vi "Dashboard Main.vi"() -> ()   [LabVIEW 2017]
uses:
  <vilib>/Utility/miscctls.llb/LVRowAndColumnTypeDef.ctl
  <vilib>/event_ctls.llb/eventvkey.ctl
  <vilib>/Rock Robotics/Network Tables/NT Read Numeric Array.vi
  <vilib>/Utility/inputDevices.llb/keyboardAcquire.vi
  <vilib>/Utility/inputDevices.llb/closeKeyboard.vi
  <vilib>/Rock Robotics/WPI/Dashboard/WPI_DashboardLogging Global.vi
panel:
  out "Key Pressed":T1(array[ring])
  out "Key Pressed as String":string
  in  "Camera Settings Right":T2={"Frame Rate"=30, "Compression"=30, "Size"=1, "DB Camera Config"=FALSE} {"Frame Rate" scale=1.0..30.0; "Compression" scale=100.0..-1.0; "Size" items=["640x480", "320x240", "160x120"]}
  in  "Camera Name Right":string(combo)="No Camera Selection"
  out "Camera Info":cluster{"Mbps LED":bool, "Mbps":dbl, "fps":dbl} {"fps" format="%#.1g"; "Mbps" format="%#.1g"}
  in  "Camera Settings":T2={"Frame Rate"=30, "Compression"=30, "Size"=1, "DB Camera Config"=FALSE} {"Frame Rate" scale=1.0..30.0; "Compression" scale=100.0..-1.0; "Size" items=["640x480", "320x240", "160x120"]}
  in  "TCP":refnum<k5>
  in  "Rec Mode":enum32{"Stop", "Record", "Playback"}(radio)
  out "Robot IP":string
  out "Image Message":string="Timeout in Camera Communications"
  in  "Dashboard Tab":T3(tab)
  in  "Select Auto":string(combo)="Select Autonomous ..."
  out "NT Connection":bool
  out "MotorChart R":cluster{"Numeric":dbl, "Numeric":dbl}(graph)
  out "MotorChart L":cluster{"Numeric":dbl, "Numeric":dbl}(graph)
  out "MotorSliders R":cluster{"MotorSlide1":dbl, "MotorSlide2":dbl} {"MotorSlide2" scale=-1.0..1.0 scale format="%#_2e"; "MotorSlide1" scale=-1.0..1.0 scale format="%#_2e"}
  out "MotorSliders L":cluster{"MotorSlide1":dbl, "MotorSlide2":dbl} {"MotorSlide2" scale=-1.0..1.0 scale format="%#_2e"; "MotorSlide1" scale=-1.0..1.0 scale format="%#_2e"}
  out "Gyro":dbl(knob) scale=0.0..360.0
  out "JS1 Z":dbl(slide) scale=-1.0..1.0 scale format="%#_2e"
  out "JS1 Graph":cluster{"X":dbl, "Y":dbl}[](graph)
  out "JS1 Buttons":T4
  out "JS2 Z":dbl(slide) scale=-1.0..1.0 scale format="%#_2e"
  out "JS2 Graph":cluster{"X":dbl, "Y":dbl}[](graph)
  out "JS2 Buttons":T4
  out "Mode":T5(ring)=enum."Auto Disabled"
  out "Camera Image Right":T6(plugin-control)
  in  "DB/String 9":string
  in  "DB/String 8":string
  in  "DB/String 7":string
  in  "DB/String 6":string
  in  "DB/String 5":string
  in  "DB/String 4":string
  in  "DB/String 3":string
  in  "DB/String 2":string
  in  "DB/String 1":string
  in  "DB/String 0":string
  in  "DB/Slider 0":dbl(slide) scale=0.0..5.0
  in  "DB/Slider 1":dbl(slide) scale=0.0..5.0
  in  "DB/Slider 2":dbl(slide) scale=0.0..5.0
  in  "DB/Slider 3":dbl(slide) scale=0.0..5.0
  out "DB/LED 3":bool
  out "DB/LED 2":bool
  out "DB/LED 1":bool
  out "DB/LED 0":bool
  in  "DB/Button 3":bool
  in  "DB/Button 2":bool
  in  "DB/Button 1":bool
  in  "DB/Button 0":bool caption="New Name"
  in  "Test Slider":dbl(slide) scale=0.0..100.0 scale format="%#_3g"
  in  "On/Off":bool caption="Solenoid"
  in  "Test Name":u16(ring) items=["Select the test to run..."]
  in  "Test Tree":string(tree)
  in  "Motor":cluster{"Value":dbl, "Enable":bool} {"Value" scale=-1.0..1.0 scale format="%#_3g"}
  out "Progress":T7 {"Test Progress" scale=0.0..100.0}
  in  "Rev/Fwd":cluster{"Forward":bool, "Reverse":bool}
  in  "Test Ring":u16(ring) items=["Monochrome", "Color"]
  out "Cmd Status":string
  in  "Execute Command":bool
  in  "Command Params":string[][](table)
  in  "Command Selection":i32(listbox)
  in  "CheckList":i32(listbox)
  out "Tree":string(tree)
  out "Camera Image":T6(plugin-control)
  out "Background":bool
  in  "Camera Name":string(combo)="No Camera Selection"
  # "HW"
  # "HW"
  # "Joysticks"
  # "Drive Motors"
  # "Front"
  # "Right"
  # "Left"
  # "Back"
  # "This tab is a great place for autonomous settings and robot-specific values.\nPlace controls and indicators inside this tab and match name to\nDashboard Variables on robot. You can also delete this comment."
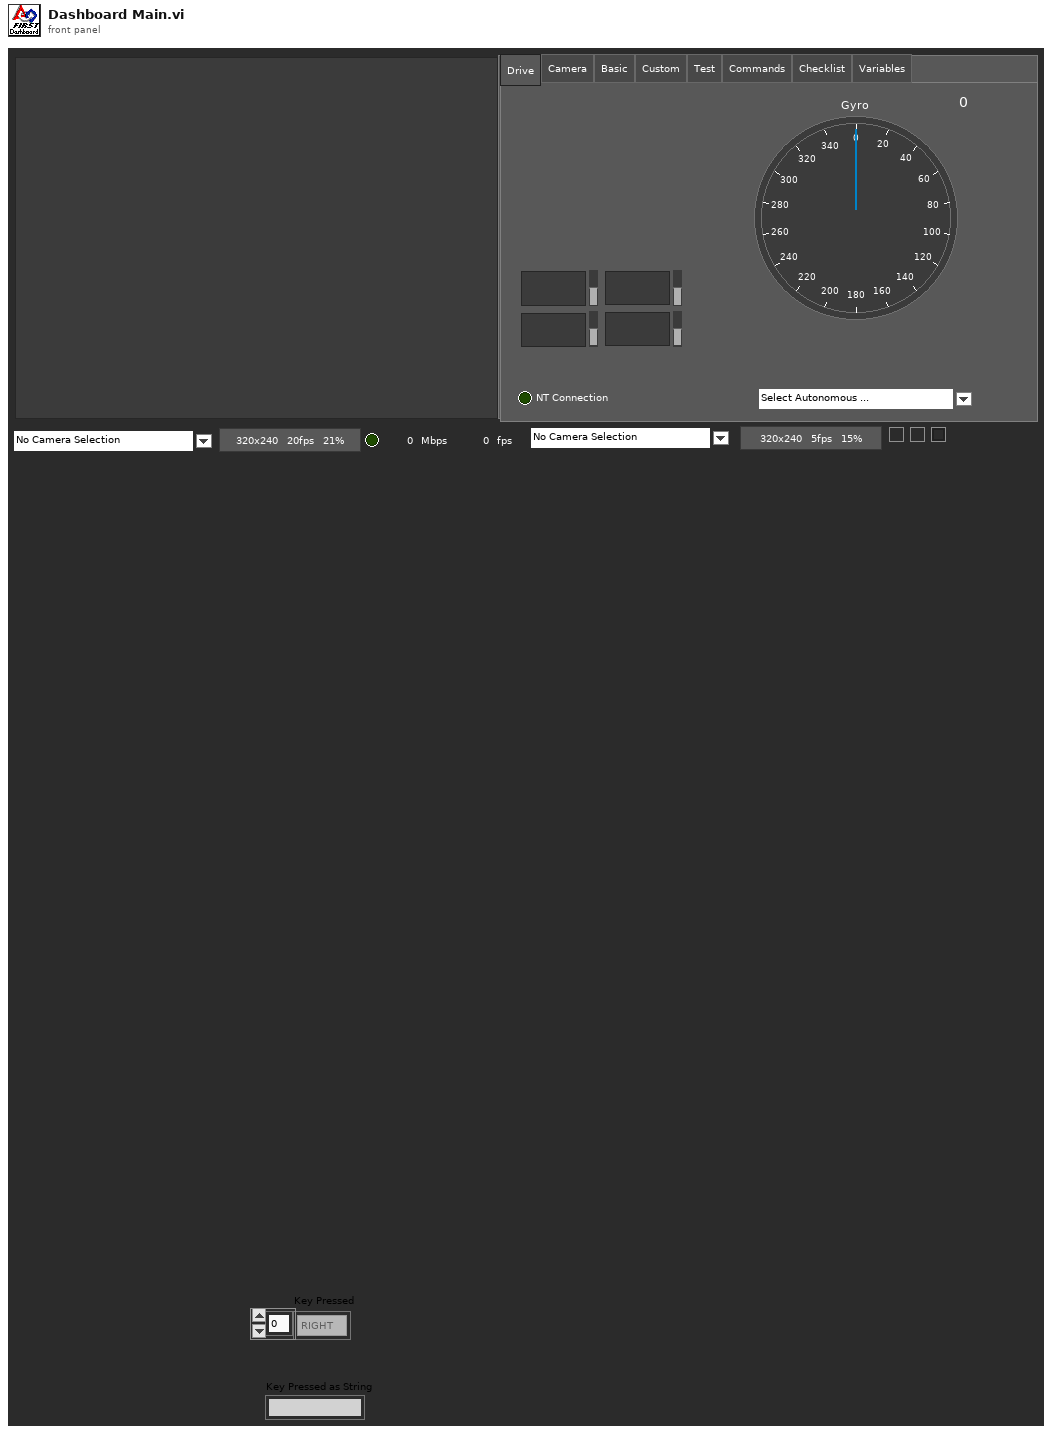
[diagram p1: front panel]
types:
  T1 = enum16{"0", "1", "2", "3", "4", "5", "6", "7", "8", "9", "A", "B", "C", "D", "E", "F", "G", "H", "I", "J", "K", "L", "M", "N", "O", "P", "Q", "R", "S", "T", "U", "V", "W", "X", "Y", "Z", "F1", "F2", "F3", "F4", "F5", "F6", "F7", "F8", "F9", "F10", "F11", "F12", "F13", "F14", "F15", "ADD", "BACK", "BACKSLASH", "CAPITAL", "COMMA", "DECIMAL", "DELETE", "DIVIDE", "DOWN", "END", "EQUALS", "ESCAPE", "GRAVE (`)", "HOME", "INSERT", "LBRACKET", "LCONTROL", "LEFT", "L ALT", "LSHIFT", "LWIN", "MINUS", "MULTIPLY", "NEXT", "NUMLOCK", "NUMPAD_0", "NUMPAD_1", "NUMPAD_2", "NUMPAD_3", "NUMPAD_4", "NUMPAD_5", "NUMPAD_6", "NUMPAD_7", "NUMPAD_8", "NUMPAD_9", "PAUSE", "PERIOD", "PRIOR (PG UP)", "RBRACKET", "RCONTROL", "RETURN", "RIGHT", "R ALT", "RSHIFT", "RWIN", "SCROLL", "SEMICOLON", "SLASH", "SPACE", "SUBTRACT", "TAB", "UP", "ENTER (num pad)", "' (quote)"}[]
  T2 = cluster{"Frame Rate":i32, "Compression":i32, "Size":u16, "DB Camera Config":bool}
  T3 = enum32{"Drive", "Camera", "Basic", "Custom", "Test", "Commands", "Checklist", "Variables"}
  T4 = cluster{bool, bool, bool, bool, bool, bool, bool, bool, bool, bool, bool, bool}
  T5 = enum8{"Tele-Op Disabled", "Tele-Op Enabled", "Auto Disabled", "Auto Enabled", "Test Disabled", "Test Enabled", "Disconnected", "No Code", "E-Stop"}
  T6 = typedef "IMAQ Image.ctl" = refnum<image>
  T7 = cluster{"Test Progress":u8, "Test Progress Text":string}
  T8 = cluster{"Save Path":path, "Interval (s)":dbl, "Keep":i32}
  T9 = typedef "Image Type" = u32
  T10 = cluster{"IDs":cluster{"RPC field ID":u16, "Unique ID":u16}, "String":string}
  T11 = cluster{"Error Strings":string, "Disable Counts":cluster{u16, u16}, "Rail Faults":cluster{u16, u16, u16}, "Robot IP":string, "DB Mode":u8, "Event Info":cluster{"Name":string, "Type":u8, "Number":u16, "Replay":u8}}
  T12 = cluster{"Storage":cluster{"Disk Free":u64, "RAM Block":u32, "RAM free":u32}, "CPU Utilization":cluster{"CPU % ISR":sgl, "CPU % Time Crit":sgl, "CPU % Timed Str":sgl, "CPU % High":sgl, "CPU % Above":sgl, "CPU % Normal":sgl, "CPU % Low":sgl}, "CAN":cluster{"% Bus Utilization":sgl, "Bus Off Cnt":u32, "TX_FIFO Full Cnt":u32, "Receive Error Cnt":u8, "Transmit Error Cnt":u8}, "HID":cluster{"HID Outputs":u32, "Rumble Low":u16, "Rumble High":u16}[]}
  T13 = cluster{"Status bits":cluster{"Test Mode":bool, "Autonomous":bool, "Enabled":bool, "Code Start":bool, "Brownout":bool, "Reserved 2":bool, "Reserved 3":bool, "E-Stop":bool}, "Code Trace":cluster{"Disabled":bool, "TeleOp":bool, "Auto":bool, "Test":bool}, "Controller Type":enum16{"unknown", "cRIO", "roboRio"}, "Code?":enum16{"unknown", "noCode", "code"}, "Battery V":dbl}
  T14 = cluster{"Control Bits":cluster{"TestMode":bool, "Autonomous":bool, "Enabled":bool, "FMS Present":bool, bool, bool, bool, "E-Stop":bool}, "Team Station ":u8, "Countdown":sgl, "Joystick Values":cluster{"Axes":dbl[], "Buttons":bool[], "POVs":i16[]}[]}
  T15 = cluster{"Axes":dbl[], "Buttons":bool[], "POVs":i16[]}[]
  T16 = enum16{"0", "1", "2", "3", "4", "5", "6", "7", "8", "9", "A", "B", "C", "D", "E", "F", "G", "H", "I", "J", "K", "L", "M", "N", "O", "P", "Q", "R", "S", "T", "U", "V", "W", "X", "Y", "Z", "F1", "F2", "F3", "F4", "F5", "F6", "F7", "F8", "F9", "F10", "F11", "F12", "F13", "F14", "F15", "ADD", "BACK", "BACKSLASH", "CAPITAL", "COMMA", "DECIMAL", "DELETE", "DIVIDE", "DOWN", "END", "EQUALS", "ESCAPE", "GRAVE (`)", "HOME", "INSERT", "LBRACKET", "LCONTROL", "LEFT", "L ALT", "LSHIFT", "LWIN", "MINUS", "MULTIPLY", "NEXT", "NUMLOCK", "NUMPAD_0", "NUMPAD_1", "NUMPAD_2", "NUMPAD_3", "NUMPAD_4", "NUMPAD_5", "NUMPAD_6", "NUMPAD_7", "NUMPAD_8", "NUMPAD_9", "PAUSE", "PERIOD", "PRIOR (PG UP)", "RBRACKET", "RCONTROL", "RETURN", "RIGHT", "R ALT", "RSHIFT", "RWIN", "SCROLL", "SEMICOLON", "SLASH", "SPACE", "SUBTRACT", "TAB", "UP", "ENTER (num pad)", "' (quote)"}
  T17 = cluster{"Axes":dbl[], "Buttons":bool[], "POVs":i16[]}
  T18 = cluster{"Buttons[0]":bool, "Buttons[1]":bool, "Buttons[2]":bool, "Buttons[3]":bool, "Buttons[4]":bool, "Buttons[5]":bool, "Buttons[6]":bool, "Buttons[7]":bool, "Buttons[8]":bool, "Buttons[9]":bool, "Buttons[10]":bool, "Buttons[11]":bool}
  T19 = cluster{"Camera Image":refnum<vi>, "Dashboard Tab":refnum<vi>, "Background":refnum<vi>, "Rec Mode":refnum<vi>, "Test Slider":refnum<vi>, "On/Off ":refnum<vi>, "Test Ring":refnum<vi>, "Rev/Fwd":refnum<vi>, "Test Name":refnum<vi>, "Motor":refnum<vi>, "Progress":refnum<vi>, "CheckList":refnum<vi>, "Tree":refnum<vi>, "Test Tree":refnum<vi>, "Command Params":refnum<vi>, "Command Selection":refnum<vi>, "Execute Command":refnum<vi>, "Cmd Status":refnum<vi>, "Camera Settings":refnum<vi>, "Camera Name":refnum<vi>, "Camera Info":refnum<vi>, "Camera Settings Right":refnum<vi>, "Camera Name Right":refnum<vi>, "Camera Image Right":refnum<vi>}
  T20 = cluster{"Camera Name":string, string, "Saved DB Images Info":cluster{"Save Path":path, "Interval (s)":dbl, "Keep":i32}}
  T21 = cluster{"Camera Name Right":string, string, "Saved DB Images Info":cluster{"Save Path":path, "Interval (s)":dbl, "Keep":i32}}
  T22 = cluster{"Operation":enum16{"Update", "Clear"}, "Color Box":u32}[]
  T23 = typedef "eventvkey.ctl" = enum16{"ASCII", "Enter", "Return", "Shift", "Ctrl", "Alt", "Cmd", "Opt", "Caps", "NumLock", "Clear", "Break", "Up", "Down", "Left", "Right", "Insert", "Delete", "Home", "End", "PageUp", "PageDown", "Escape", "Help", "Pause", "ScrollLock", "F1", "F2", "F3", "F4", "F5", "F6", "F7", "F8", "F9", "F10", "F11", "F12", "F13", "F14", "F15", "F16", "F17", "F18", "F19", "F20", "F21", "F22", "F23", "F24", "Play", "VolumeUp", "VolumeDown", "Mute", "Two Byte Char"}
  T24 = cluster{"Image Size":bool, "Image Type":bool, "Pixel Value":bool, "ROI Information":bool, "Zoom Factor":bool}
  T25 = cluster{"Operation":enum16{"Update", "Clear"}, "Color Box":u32}
  T26 = typedef "LVRowAndColumnTypeDef.ctl" = cluster{"Row":i32, "Column":i32}
  T27 = cluster{"Shift":bool, "Ctrl":bool, "Alt":bool, "Cmd":bool, "Opt":bool}
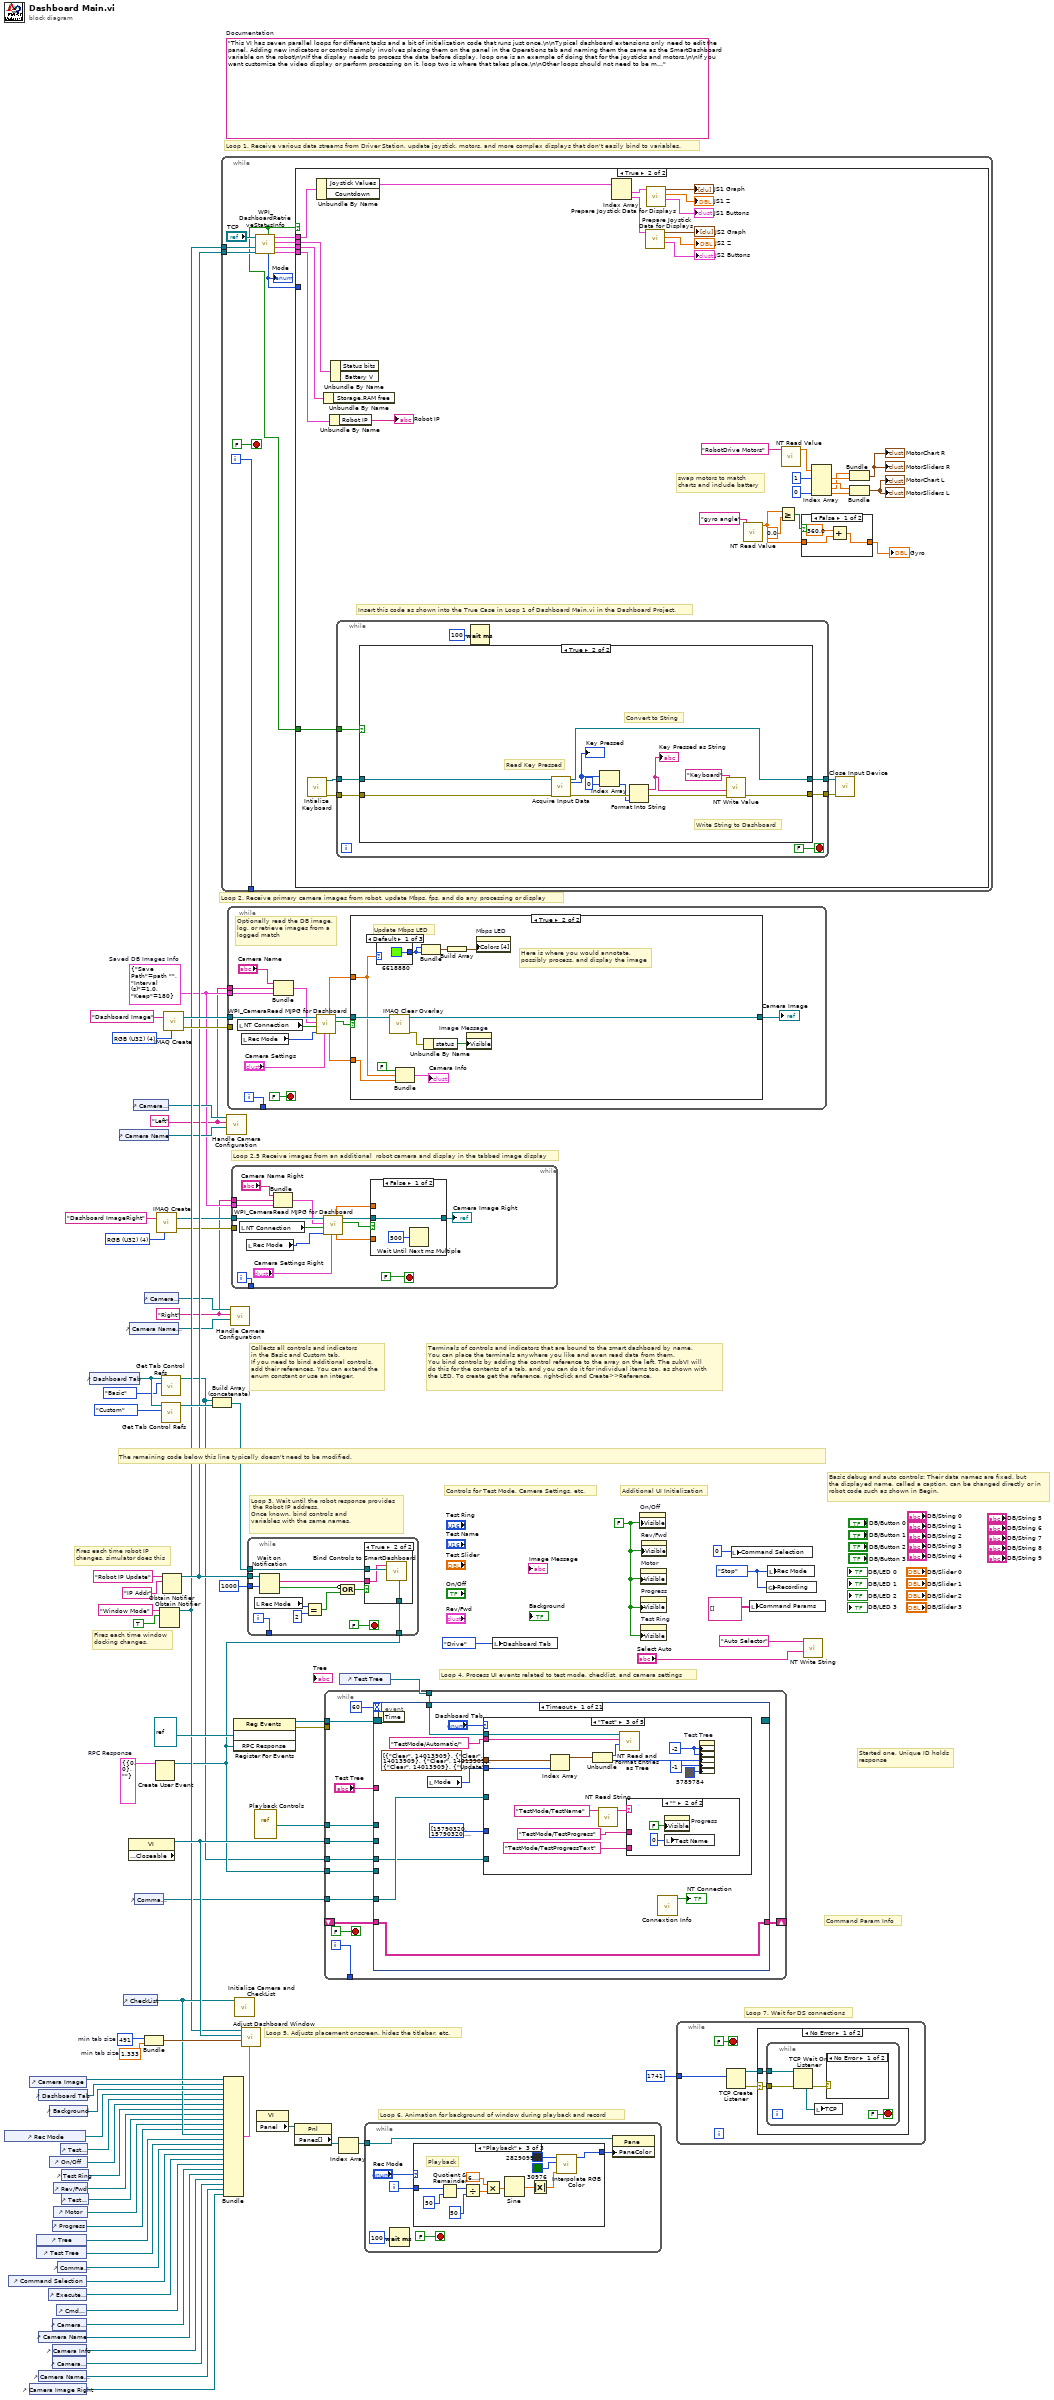
[diagram p0: block diagram]
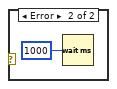
[diagram p3: hidden frame]
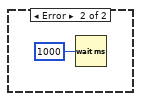
[diagram p4: hidden frame]
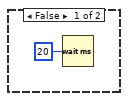
[diagram p5: hidden frame]
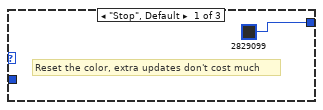
[diagram p8: hidden frame]
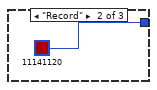
[diagram p9: hidden frame]
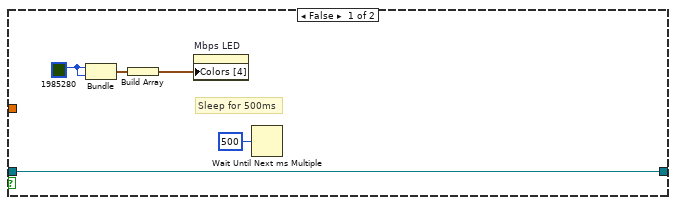
[diagram p11: hidden frame]
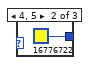
[diagram p12: hidden frame]
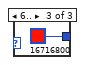
[diagram p13: hidden frame]
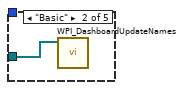
[diagram p15: hidden frame]
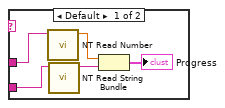
[diagram p16: hidden frame]
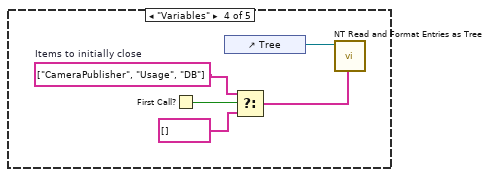
[diagram p17: hidden frame]
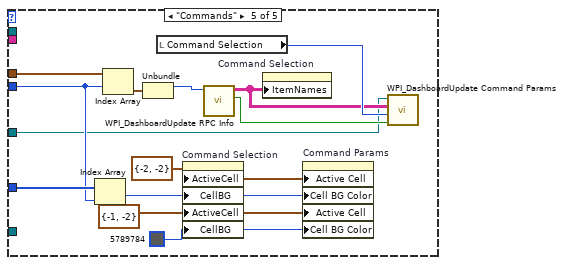
[diagram p18: hidden frame]
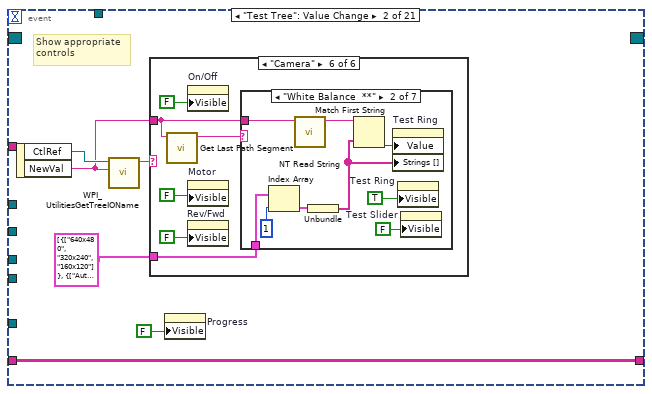
[diagram p19: hidden frame]
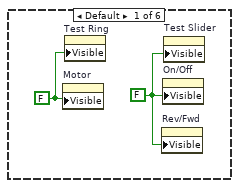
[diagram p20: hidden frame]
diagram:
  w3 = T8 {"Save Path"=path "", "Interval (s)"=1.0, "Keep"=180}  # Saved DB Images Info
  w2 = "Right"
  w1 = "Left"
  w13 = T9 4 items=["Grayscale (U8)", "Grayscale (I16)", "Grayscale (SGL)", "Complex (CSG)", "RGB (U32)", "HSL (U32)", "RGB (U64)"] ("Image Type")
  w29 = T10 {"IDs"={"RPC field ID"=0, "Unique ID"=0}, "String"=""}  # RPC Response
  w52 = 491  # min tab size
  w51 = 1.333  # min tab size
  w59 = enum32{"Stop", "Record", "Playback"}."Stop" ("Rec Mode")
  w36 = FALSE ("Visible")
  (unwired) "This VI has seven parallel loops for different tasks and a bit of initialization code that runs just once.\n\nTypical dashboard extensions only need to edit the panel. Adding new indicators or controls simply involves placing them on the panel in the Operations tab and naming them the same as the SmartDashboard variable on the robot\n\nIf the display needs to process the data before display, loop one is an example of doing that for the joysticks and motors.\n\nIf you want customize the video display or perform processing on it, loop two is where that takes place.\n\nOther loops should not need to be modified. They are pretty standard, and document the task they perform."  # Documentation
  w76 = T9 4 items=["Grayscale (U8)", "Grayscale (I16)", "Grayscale (SGL)", "Complex (CSG)", "RGB (U32)", "HSL (U32)", "RGB (U64)"] ("Image Type")
  # "Loop 2.5 Receive images from an additional  robot camera and display in the tabbed image display"
  # "Command Param Info"
  # "Started one, Unique ID holds\nresponse"
  # "Loop 7. Wait for DS connections"
  # "Basic debug and auto controls: Their data names are fixed, but\nthe displayed name, called a caption, can be changed directly or in\nrobot code such as shown in Begin."
  # "Controls for Test Mode, Camera Settings, etc."
  # "Additional UI Initialization"
  # "Loop 6. Animation for background of window during playback and record"
  # "Fires each time robot IP\nchanges, simulator does this"
  # "Fires each time window\ndocking changes."
  # "Collects all controls and indicators\nin the Basic and Custom tab.\nIf you need to bind additional controls,\nadd their references. You can extend the\nenum constant or use an integer."
  # "The remaining code below this line typically doesn't need to be modified."
  # "Loop 4. Process UI events related to test mode, checklist, and camera settings"
  # "Terminals of controls and indicators that are bound to the smart dashboard by name.\nYou can place the terminals anywhere you like and even read data from them.\nYou bind controls by adding the control reference to the array on the left. The subVI will\ndo this for the contents of a tab, and you can do it for individual items too, as shown with\nthe LED. To create get the reference, right-click and Create>>Reference."
  # "Loop 3. Wait until the robot response provides\n the Robot IP address.\nOnce known, bind controls and\nvariables with the same names."
  # "Loop 5. Adjusts placement onscreen, hides the titlebar, etc."
  # "Loop 1. Receive various data streams from Driver Station, update joystick, motors, and more complex displays that don't easily bind to variables."
  # "Loop 2. Receive primary camera images from robot, update Mbps, fps, and do any processing or display"
  n1 = control-ref of="Rec Mode"() -> (w42:refnum<vi>)
  n2 = control-ref of="Command Selection"() -> (w28:refnum<vi>)
  n3 = control-ref of="Camera Image Right"() -> (w6:refnum<vi>)
  n4 = control-ref of="Camera Image"() -> (w54:refnum<vi>)
  n5 = control-ref of="Tree"() -> (w46:refnum<vi>)
  n6 = control-ref of="Test Tree"() -> (w45:refnum<vi>)
  n7 = control-ref of="Dashboard Tab"() -> (w53:refnum<vi>)
  n8 = control-ref of="Camera Name"() -> (w19:refnum<vi>)
  n9 = control-ref of="Camera Name Right"() -> (w7:refnum<vi>)
  n10 = control-ref of="Execute Command"() -> (w30:refnum<vi>)
  n11 = control-ref of="Background"() -> (w49:refnum<vi>)
  n12 = control-ref of="On/Off"() -> (w40:refnum<vi>)
  n13 = control-ref of="Progress"() -> (w37:refnum<vi>)
  n14 = control-ref of="Camera Settings"() -> (w20:refnum<vi>)
  n15 = control-ref of="Camera Info"() -> (w18:refnum<vi>)
  n16 = control-ref of="Camera Settings Right"() -> (w8:refnum<vi>)
  n17 = control-ref of="Rev/Fwd"() -> (w38:refnum<vi>)
  n18 = control-ref of="Motor"() -> (w43:refnum<vi>)
  n19 = control-ref of="Cmd Status"() -> (w24:refnum<vi>)
  n20 = control-ref of="Command Params"() -> (w31:refnum<vi>)
  n21 = control-ref of="Test Slider"() -> (w41:refnum<vi>)
  n22 = control-ref of="Test Ring"() -> (w39:refnum<vi>)
  n23 = control-ref of="Test Name"() -> (w44:refnum<vi>)
  n24 = control-ref of="Dashboard Tab"() -> (w57:refnum<vi>)
  n25 = control-ref of="Camera Name"() -> (w21:refnum<vi>)
  n26 = control-ref of="CheckList"() -> (w47:refnum<vi>)
  n27 = property class="VI" props=["Front Panel.Closeable"]() -> (reference out=w58:refnum<vi>)  [unwired: 2 in, 2 out]
  n28 = control-ref of="Camera Name Right"() -> (w9:refnum<vi>)
  n29 = control-ref of="Camera Settings"() -> (w22:refnum<vi>)
  n30 = control-ref of="Command Params"() -> (w23:refnum<vi>)
  n31 = control-ref of="Camera Settings Right"() -> (w10:refnum<vi>)
  n32 = Bundle("min tab size"=w52, "min tab size"=w51) -> (w50:cluster{"min tab size":i32, "min tab size":dbl})  [unwired: 1 in]
  n33 = Create User Event(user event datatype=w29) -> (user event=w25:refnum<user-event>)  [unwired: 1 in, 1 out]
  n34 = call "IMAQ Create"("Image Name"="Dashboard ImageRight", "Image Type"=w13) -> ("New Image"=w12:T6, "error out"=w11:errorcluster)  [unwired: 2 in, 1 out]
  n35 = Obtain Notifier(name (unnamed)="Window Mode", notification data type=TRUE) -> (notifier out=w34:refnum<notifier>)  [unwired: 2 in, 2 out]
  n36 = call <vilib>:"Get Tab Control Refs.vi"("Page Index"=T3."Basic" ("Dashboard Tab"), "TabControl in"=w57) -> ("ControlsOnPage"=w17:refnum<vi>[])  [unwired: 9 in]
  n37 = call <vilib>:"Get Tab Control Refs.vi"("Page Index"=T3."Custom" ("Dashboard Tab"), "TabControl in"=w57) -> ("ControlsOnPage"=w56:refnum<vi>[])  [unwired: 9 in]
  n38 = Obtain Notifier(name (unnamed)="Robot IP Update", notification data type="IP Addr" ("name (unnamed)")) -> (notifier out=w35:refnum<notifier>)  [unwired: 2 in, 2 out]
  n39 = call "IMAQ Create"("Image Name"="Dashboard Image", "Image Type"=w76) -> ("New Image"=w74:T6, "error out"=w73:errorcluster)  [unwired: 2 in, 1 out]
  n40 = Build Array (concatenate)(w17, w56) -> (w55:refnum<vi>[])
  n41 = while {
    tunnel: [w86] -> _
    tunnel: w35 -> [w81]
    tunnel: w34 -> [w78]
    i -> [w86]
    stop <- FALSE stop-if-true
    n42 = call <vilib>:"WPI_DashboardRetrieveStatusInfo.vi"("Binding Refnum"=w81, "Window Mode Notifier"=w78, "TCP Cnx"="TCP") -> ("Power and Errors"=w82:T11, "Robot Metrics"=w84:T12, "Status Info"=w85:T13, "Control Info"=w83:T14, "Robot Mode"=w80:T5, "Process?"=w77:bool)  [unwired: 3 in]
    "Mode" <- w80
    n43 = case shown="True" w77 {
      tunnel: w85 -> [_ w122]
      tunnel: w84 -> [_ w121]
      tunnel: w83 -> [_ w120]
      tunnel: w82 -> [_ w119]
      tunnel: w80 -> [_ _]
      tunnel: w77 -> [_ w89]
      frame False {
        n44 = Wait (ms)(milliseconds to wait=u32 20) -> ()  [unwired: 1 out]
      }
      frame True {
        # "Insert this code as shown into the True Case in Loop 1 of Dashboard Main.vi in the Dashboard Project."
        # "swap motors to match\ncharts and include battery"
        n45 = call <vilib>:"Intialize Keyboard.vi"() -> ("error out"=w92:errorcluster, "device ID"=w93:refnum<k1>)  [unwired: 10 in]
        n46 = Unbundle By Name(w120) -> ("Joystick Values"=w110:T15)  [unwired: 1 out]
        n47 = Unbundle By Name(w121) -> ()  [unwired: 1 out]
        n48 = Unbundle By Name(w119) -> ("Robot IP"=→"Robot IP":string)
        n49 = Unbundle By Name(w122) -> ()  [unwired: 2 out]
        n50 = while {
          tunnel: w93 -> [w129]
          tunnel: w92 -> [w128]
          tunnel: [w127] -> w91
          tunnel: [w126] -> w90
          tunnel: w89 -> [w125]
          stop <- FALSE stop-if-true
          n51 = case shown="True" w125 {
            tunnel: w129 -> [_ w136]
            tunnel: w128 -> [_ w135]
            tunnel: [_ w132] -> w127
            tunnel: [_ w134] -> w126
            frame False {
            }
            frame True {
              # "Write String to Dashboard"
              # "Convert to String"
              # "Read Key Pressed"
              n52 = call-poly <vilib>:"Acquire Input Data.vi"("device ID"=w136, "error in (no error)"=w135) -> ("device ID"=w134:refnum<k1>, "keys pressed"=w138:T1, "error out"=w140:errorcluster)  [unwired: 15 in]
              "Key Pressed" <- w138
              n53 = Index Array(array=w138, index=0) -> (element=w139:T16)
              n54 = Format Into String(error in=w140, w139) -> (resulting string=w131:string, error out=w133:errorcluster)  [unwired: 2 in]
              "Key Pressed as String" <- w131
              n55 = call-poly <vilib>:"NT Write Value.vi"("error in"=w133, "String"=w131, "Name"="Keyboard") -> ("error out"=w132:errorcluster)  [unwired: 8 in]
            }
          }
          n56 = Wait (ms)(milliseconds to wait=u32 100) -> ()  [unwired: 1 out]
        }
        n57 = Index Array(array=w110) -> (element #1=w109:T17, element #2=w105:T17)  [unwired: 2 in]
        n58 = call "Prepare Joystick Data for Displays.vi"("Joystick Values"=w105) -> ("Buttons"=→"JS2 Buttons":T18, "Z Axis"=→"JS2 Z":dbl, "Cartesian Data"=→"JS2 Graph":cluster{"X axis":dbl, "X axis":dbl}[])  [unwired: 8 in]
        n59 = call "Prepare Joystick Data for Displays.vi"("Joystick Values"=w109) -> ("Buttons"=→"JS1 Buttons":T18, "Z Axis"=→"JS1 Z":dbl, "Cartesian Data"=→"JS1 Graph":cluster{"X axis":dbl, "X axis":dbl}[])  [unwired: 8 in]
        n60 = call-poly <vilib>:"NT Read Value.vi"("Name"="gyro angle") -> ("Numeric"=w94:dbl)  [unwired: 9 in, 1 out]
        n61 = Greater Or Equal?(x=w94, y=0.0) -> (x >= y?=w96:bool)
        n62 = call-poly <vilib>:"NT Read Value.vi"("Name"="RobotDrive Motors") -> ("Numeric Array"=w100:dbl[])  [unwired: 9 in, 1 out]
        n63 = case shown="False" w96 {
          tunnel: [w141 w144] -> w95
          tunnel: w94 -> [w142 w144]
          frame False {
            n64 = Add(x=360.0, y=w142) -> (x+y=w141:dbl)
          }
          frame True {
          }
        }
        "Gyro" <- w95
        n65 = Index Array(array=w100, index #1=1, index #4=0) -> (element #1=w114:dbl, element #2=w115:dbl, element #3=w113:dbl, element #4=w118:dbl)  [unwired: 2 in]
        n66 = call-poly <vilib>:"Close Input Device.vi"("error in (no error)"=w91, "device ID"=w90) -> ()  [unwired: 8 in, 1 out]
        n67 = Bundle("Numeric"=w113, "Numeric"=w114) -> (→"MotorChart R" →"MotorSliders R":cluster{"Numeric":dbl, "Numeric":dbl})  [unwired: 1 in]
        n68 = Bundle("Numeric"=w115, "Numeric"=w118) -> (→"MotorChart L" →"MotorSliders L":cluster{"Numeric":dbl, "Numeric":dbl})  [unwired: 1 in]
      }
    }
  }
  n69 = Bundle("Camera Image"=w54, "Dashboard Tab"=w53, "Background"=w49, "Rec Mode"=w42, "Test Slider"=w41, "On/Off"=w40, "Test Ring"=w39, "Rev/Fwd"=w38, "Test Name"=w44, "Motor"=w43, "Progress"=w37, "CheckList"=w47, "Tree"=w46, "Test Tree"=w45, "Command Params"=w31, "Command Selection"=w28, "Execute Command"=w30, "Cmd Status"=w24, "Camera Settings"=w20, "Camera Name"=w19, "Camera Info"=w18, "Camera Settings Right"=w8, "Camera Name Right"=w7, "Camera Image Right"=w6) -> (w48:T19)  [unwired: 1 in]
  n70 = call "Handle Camera Configuration.vi"("CameraNameRef"=w21, "Display Name"=w1, "ClusterRef"=w22) -> ()  [unwired: 9 in]
  n71 = while {
    tunnel: w74 -> [w157]
    tunnel: w73 -> [_]
    tunnel: [w158] -> _
    tunnel: w3 -> [w148]
    tunnel: w1 -> [w145]
    i -> [w158]
    stop <- FALSE stop-if-true
    # "Optionally read the DB image,\nlog, or retrieve images from a\nlogged match"
    n72 = local read "NT Connection"() -> (w149:bool)
    n73 = local read "Rec Mode"() -> (w153:enum32{"Stop", "Record", "Playback"})
    n74 = Bundle("Camera Name"="Camera Name", w145, "Saved DB Images Info"=w148) -> (w147:T20)  [unwired: 1 in]
    n75 = call <vilib>:"WPI_CameraRead MJPG for Dashboard.vi"("Camera Settings"="Camera Settings", "Rec Mode"=w153, "NT Connection"=w149, "Capture Info"=w147, "Refnum in"=w157) -> ("Active"=w155:bool, "Refnum out"=w156:T6, "FPS"=w154:dbl, "Bandwidth (Mbps)"=w152:dbl)  [unwired: 3 in]
    n76 = case shown="True" w155 {
      tunnel: w156 -> [w160 w171]
      tunnel: w152 -> [_ w168]
      tunnel: w154 -> [_ w169]
      tunnel: [w160 w165] -> w150
      frame False {
        w162 = u32 1985280 ("Color Box")
        # "Sleep for 500ms"
        n77 = Bundle("Color Box"=w162, "Color Box"=w162) -> (w163:cluster{"Color Box":u32, "Color Box":u32})  [unwired: 1 out]
        n78 = Build Array(w163) -> (w161:cluster{"Color Box":u32, "Color Box":u32}[])
        n79 = property on="Mbps LED" class="Bool (strict)"("Colors [4]"=w161) -> ()  [unwired: 2 in, 2 out]
        n80 = Wait Until Next ms Multiple(millisecond multiple=u32 500) -> ()  [unwired: 1 out]
      }
      frame True {
        # "Here is where you would annotate,\npossibly process, and display the image"
        # "Update Mbps LED"
        n81 = case shown="Default" w168 {
          tunnel: [u32 6618880 ("Color Box") u32 16776722 ("Color Box") u32 16716800 ("Color Box")] -> w172
          frame Default {
          }
          frame 4, 5 {
          }
          frame 6.. {
          }
        }
        n82 = call "IMAQ Clear Overlay"("Image"=w171) -> ("error out"=w174:errorcluster, "Image Out"=w165:T6)  [unwired: 2 in, 7 out]
        n83 = Bundle(FALSE, "Bandwidth (Mbps)"=w168, "FPS"=w169) -> (→"Camera Info":cluster{bool, "Bandwidth (Mbps)":dbl, "FPS":dbl})  [unwired: 1 in]
        n84 = Bundle("Color Box"=w172, "Color Box"=w172) -> (w173:cluster{"Color Box":u32, "Color Box":u32})  [unwired: 1 out]
        n85 = Unbundle By Name(w174) -> ("status"=w175:bool)
        n86 = Build Array(w173) -> (w170:cluster{"Color Box":u32, "Color Box":u32}[])
        n87 = property on="Image Message" class="Str"("Visible"=w175) -> ()  [unwired: 2 in, 2 out]
        n88 = property on="Mbps LED" class="Bool (strict)"("Colors [4]"=w170) -> ()  [unwired: 2 in, 2 out]
      }
    }
    "Camera Image" <- w150
  }
  n89 = call "Handle Camera Configuration.vi"("CameraNameRef"=w9, "Display Name"=w2, "ClusterRef"=w10) -> ()  [unwired: 9 in]
  n90 = while {
    tunnel: w12 -> [w193]
    tunnel: w11 -> [_]
    tunnel: [w188] -> _
    tunnel: w3 -> [w182]
    tunnel: w2 -> [w179]
    i -> [w188]
    stop <- FALSE stop-if-true
    n91 = local read "NT Connection"() -> (w183:bool)
    n92 = local read "Rec Mode"() -> (w192:enum32{"Stop", "Record", "Playback"})
    n93 = Bundle("Camera Name Right"="Camera Name Right", w179, "Saved DB Images Info"=w182) -> (w181:T21)  [unwired: 1 in]
    n94 = call <vilib>:"WPI_CameraRead MJPG for Dashboard.vi"("Camera Settings"="Camera Settings Right", "Rec Mode"=w192, "NT Connection"=w183, "Capture Info"=w181, "Refnum in"=w193) -> ("Active"=w187:bool, "Refnum out"=w190:T6, "FPS"=w185:dbl, "Bandwidth (Mbps)"=w186:dbl)  [unwired: 3 in]
    n95 = case shown="False" w187 {
      tunnel: w190 -> [w194 w196]
      tunnel: w186 -> [_ _]
      tunnel: w185 -> [_ _]
      tunnel: [w194 w196] -> w184
      frame False {
        n96 = Wait Until Next ms Multiple(millisecond multiple=u32 500) -> ()  [unwired: 1 out]
      }
      frame True {
      }
    }
    "Camera Image Right" <- w184
  }
  n97 = register-events(refnum<vi> refnum, w25) -> (reference out=w63:refnum<event-registration>, error out=w62:errorcluster)  [unwired: 2 in]
  n98 = call "Initialize Camera and CheckList.vi"("ListBox in"=w47) -> ()  [unwired: 11 in]
  n99 = call "Adjust Dashboard Window.vi"("Sizing Refnums"=w48, "Size Constraints"=w50, "VI"=w58, "WIn Mode"=w34) -> ()  [unwired: 8 in]
  n100 = while {
    tunnel: w55 -> [w208]
    tunnel: w35 -> [w206]
    tunnel: [w204] -> _
    tunnel: u32 1000 ("milliseconds to wait") -> [w203]
    tunnel: w25 -> [w197]
    i -> [w204]
    stop <- FALSE stop-if-true
    n101 = local read "Rec Mode"() -> (w199:enum32{"Stop", "Record", "Playback"})
    n102 = Wait on Notification(notifier=w206, timeout in ms (-1)=w203) -> (notification=w205:string, timed out?=w201:bool)  [unwired: 2 in, 2 out]
    n103 = Equal?(x=w199, y=u16 2 ("Rec Mode")) -> (x = y?=w200:bool)
    n104 = Compound Arithmetic op=OR(invert w201, w200) -> (w202:bool)
    n105 = case shown="True" w202 {
      tunnel: w208 -> [_ w211]
      tunnel: w205 -> [_ w210]
      tunnel: w197 -> [_ w209]
      frame False {
      }
      frame True {
        n106 = call <vilib>:"Bind Controls to SmartDashboard.vi"("RPC ref"=w209, "Bound Control Refs"=w211, "Server IP Address"=w210) -> ()  [unwired: 9 in]
      }
    }
  }
  n107 = vi-ref "Playback Controls.vi"() -> (w64:refnum<vi>)
  n108 = property class="VI"() -> ("Panel"=w66:refnum<vi>)  [unwired: 2 in, 2 out]
  n109 = property class="Pnl"(reference=w66) -> ("Panes[]"=w67:refnum<vi>[])  [unwired: 1 in, 2 out]
  n110 = Index Array(array=w67) -> (element=w65:refnum<vi>)  [unwired: 1 in]
  n111 = control-ref of="Test Tree"() -> (w68:refnum<vi>)
  n112 = while {
    tunnel: [w221] -> _
    tunnel: w68 -> [w220]
    tunnel: w64 -> [w219]
    tunnel: w63 -> [w218]
    tunnel: w62 -> [_]
    tunnel: w58 -> [w217]
    tunnel: w25 -> [w216]
    tunnel: w23 -> [w215]
    shift-right: [w214] -> _
    shift-left: _ -> [w213]
    tunnel: w17 -> [w212]
    i -> [w221]
    stop <- FALSE stop-if-true
    n113 = event shown="[0] Timeout" {
      selector: w218 -> [_ _ _ _ _ _ _ _ _ _ _ _ _ _ _ _ _ _ _ _ _]
      dyn-events: [_ _ _ _ _ _ _ _ _ _ _ _ _ _ _ _ w481 _ _ _ _] -> _
      timeout: u32 60 ("milliseconds to wait") -> [_ _ _ _ _ _ _ _ _ _ _ _ _ _ _ _ _ _ _ _ _]
      tunnel: w220 -> [w233 _ _ _ _ _ _ _ _ _ _ _ _ _ _ _ _ _ _ _ _]
      tunnel: "Test Tree" -> [_ _ _ _ _ _ _ _ _ _ _ w448 w456 w458 w462 w470 _ _ _ _ _]
      tunnel: w219 -> [_ _ _ _ _ _ _ _ _ _ _ _ _ _ _ _ w483 _ w501 _ _]
      tunnel: w217 -> [_ _ _ _ _ _ _ _ _ _ _ _ _ _ _ _ w479 _ _ _ _]
      tunnel: w216 -> [_ _ _ _ _ _ _ _ _ _ _ _ _ _ _ _ w477 _ _ _ _]
      tunnel: w215 -> [w228 _ _ _ _ _ w399 _ _ _ _ _ _ _ _ _ _ _ _ _ _]
      tunnel: [w227 w276 w378 w383 w392 w396 w397 w406 w416 w423 w435 w447 w454 w457 w461 w469 w476 w496 w498 w502 w515] -> w214
      tunnel: w213 -> [w227 w276 w378 w383 w392 w396 w397 _ _ w423 w435 w447 w454 w457 w461 w469 w476 w496 w498 w502 w515]
      tunnel: w212 -> [w225 _ _ _ _ _ _ _ _ _ _ _ _ _ _ _ _ _ _ _ _]
      event Timeout {
        n114 = event-data() -> ()  [unwired: 1 in, 1 out]
        n115 = local read "Mode"() -> (w230:T5)
        n116 = case shown="\"Test\"" "Dashboard Tab" {
          tunnel: w233 -> [_ _ w249 _ _]
          tunnel: "TestMode/Automatic/" ("Name Pattern") -> [_ _ w248 _ _]
          tunnel: T22 [{"Operation"=enum."Clear", "Color Box"=14013909}, {"Operation"=enum."Clear", "Color Box"=14013909}, {"Operation"=enum."Clear", "Color Box"=14013909}, {"Operation"=enum."Clear", "Color Box"=14013909}, {"Operation"=enum."Update", "Color Box"=14013909}, {"Operation"=enum."Update", "Color Box"=16777215}, {"Operation"=enum."Clear", "Color Box"=14013909}, {"Operation"=enum."Clear", "Color Box"=14013909}, {"Operation"=enum."Clear", "Color Box"=14013909}] -> [_ _ w241 _ w269]
          tunnel: w230 -> [_ _ w240 _ w268]
          tunnel: u32[] [15790320, 15790320, 15790320, 15790320, 16777215, 16777215, 15790320, 15790320, 15790320] -> [_ _ _ _ w274]
          tunnel: w228 -> [_ _ _ _ w262]
          tunnel: w225 -> [_ w235 _ _ _]
          frame "Custom", Default {
          }
          frame "Basic" {
            n117 = call <vilib>:"WPI_DashboardUpdateNames.vi"("Controls on Tab"=w235) -> ()  [unwired: 11 in]
          }
          frame "Test" {
            w247 = -2 ("Active Item:Row Number")
            n118 = Index Array(array=w241, index=w240) -> (element=w242:T25)
            n119 = Unbundle(w242) -> ("Operation"=w243:enum16{"Update", "Clear"}, "Color Box"=w244:u32)
            n120 = call <vilib>:"NT Read String.vi"("Name"="TestMode/TestName") -> ("String"=w238:string)  [unwired: 9 in, 1 out]
            n121 = call <vilib>:"NT Read and Format Entries as Tree.vi"("Operation"=w243, "Name Pattern"=w248, "Tree Refnum"=w249) -> ()  [unwired: 7 in, 2 out]
            n122 = case shown="\"\"" w238 {
              tunnel: "TestMode/TestProgress" ("Name") -> [w251 _]
              tunnel: "TestMode/TestProgressText" ("Name") -> [w250 _]
              frame Default {
                n123 = call <vilib>:"NT Read Number.vi"("Name"=w251) -> ("Numeric"=w252:dbl)  [unwired: 9 in, 1 out]
                n124 = call <vilib>:"NT Read String.vi"("Name"=w250) -> ("String"=w253:string)  [unwired: 9 in, 1 out]
                n125 = Bundle("Numeric"=w252, "String"=w253) -> (→"Progress":cluster{"Numeric":dbl, "String":string})  [unwired: 1 in]
              }
              frame "" {
                n126 = property on="Progress" class="Clust (strict)"("Visible"=FALSE) -> ()  [unwired: 2 in, 2 out]
                n127 = local write "Test Name"(u16 0) -> ()
              }
            }
            n128 = property on="Test Tree" class="Tree (strict)"("Active Item Row Number"=w247, "ActiveColNum"=w247, "CellBG"=w244, "Active Item Row Number"=-1 ("Active Item:Row Number"), "CellBG"=u32 5789784 ("Color Box")) -> ()  [unwired: 2 in, 2 out]
          }
          frame "Variables" {
            w259 = string[] ["CameraPublisher", "Usage", "DB"]  # Items to initially close
            n129 = First Call?() -> (First Call?: T/F=w260:bool)
            n130 = control-ref of="Tree"() -> (w261:refnum<vi>)
            n131 = Select(t=w259, s=w260, f=string[] []) -> (s? t:f=w257:string[])
            n132 = call <vilib>:"NT Read and Format Entries as Tree.vi"("Tags to  Close"=w257, "Tree Refnum"=w261) -> ()  [unwired: 8 in, 2 out]
          }
          frame "Commands" {
            w270 = u32 5789784 ("Color Box")
            w271 = T26 {"Row"=-1, "Column"=-2} ("Active Cell:Active Cell")
            w273 = T26 {"Row"=-2, "Column"=-2} ("Active Cell:Active Cell")
            n133 = Index Array(array=w274, index=w268) -> (element=w272:u32)
            n134 = Index Array(array=w269, index=w268) -> (element=w267:T25)
            n135 = Unbundle(w267) -> ("Operation"=w266:enum16{"Update", "Clear"})  [unwired: 1 out]
            n136 = local read "Command Selection"() -> (w265:i32)
            n137 = property on="Command Selection" class="MCListbox (strict)"("ActiveCell"=w273, "CellBG"=w272, "ActiveCell"=w271, "CellBG"=w270) -> ()  [unwired: 2 in, 2 out]
            n138 = call <vilib>:"WPI_DashboardUpdate RPC Info.vi"("Operation"=w266) -> ("update"=w264:bool, "commands"=w263:string[][])  [unwired: 9 in]
            n139 = property on="Command Selection" class="MCListbox (strict)"("ItemNames"=w263) -> ()  [unwired: 2 in, 2 out]
            n140 = property on="Command Params" class="Tbl (strict)"("Active Cell"=w273, "Cell BG Color"=w272, "Active Cell"=w271, "Cell BG Color"=w270) -> ()  [unwired: 2 in, 2 out]
            n141 = call <vilib>:"WPI_DashboardUpdate Command Params.vi"("Update"=w264, "NewVal"=w265, "Commands"=w263, "Param Tbl"=w262) -> ()  [unwired: 7 in, 1 out]
          }
        }
        n142 = call <vilib>:"Connextion Info.vi"() -> ("Connected"=→"NT Connection":bool)  [unwired: 10 in, 1 out]
      }
      event "Test Tree": Value Change {
        # "Show appropriate\ncontrols"
        n143 = event-data() -> ("CtlRef"=w279:refnum<vi>, "NewVal"=w277:string)  [unwired: 1 in]
        n144 = call <vilib>:"WPI_UtilitiesGetTreeIOName.vi"("NewVal"=w277, "TreeControl in"=w279) -> ("I/O Name"=w280:string)  [unwired: 9 in]
        n145 = case shown="\"Camera\"" w280 {
          selector: w280 -> [_ w287 _ w309 w318 _]
          tunnel: w277 -> [_ _ w306 w308 _ w325]
          tunnel: cluster{string[]}[] [{["640x480", "320x240", "160x120"]}, {["Auto", "Fixed indoor", "Fixed outdoor 1", "Fixed outdoor 2", "Fixed fluorescent 1", "Fixed fluorescent 2", "Hold current"]}, {["Auto", "Flicker-free 50 Hz", "Flicker-free 60 Hz", "Hold current"]}, {["None", "Prioritize frame rate", "Prioritize image quality"]}, {["Monochrome", "Color"]}] -> [_ _ _ _ _ w324]
          frame Default {
            w282 = FALSE ("Visible")
            w281 = FALSE ("Visible")
            n146 = property on="Motor" class="Clust (strict)"("Visible"=w281) -> ()  [unwired: 2 in, 2 out]
            n147 = property on="Test Ring" class="Ring (strict)"("Visible"=w281) -> ()  [unwired: 2 in, 2 out]
            n148 = property on="Rev/Fwd" class="Clust (strict)"("Visible"=w282) -> ()  [unwired: 2 in, 2 out]
            n149 = property on="On/Off" class="Bool (strict)"("Visible"=w282) -> ()  [unwired: 2 in, 2 out]
            n150 = property on="Test Slider" class="Slide (strict)"("Visible"=w282) -> ()  [unwired: 2 in, 2 out]
          }
          frame "Analog Out", "Motor", "PWM" {
            w288 = FALSE ("Visible")
            n151 = case shown="\"Analog Out\"" w287 {
              tunnel: [1.0 ("Value") -1.0 ("Value") 0.0 ("Value")] -> w286
              tunnel: [255.0 ("Value") 1.0 ("Value") 5.0 ("Value")] -> w285
              tunnel: [128.0 ("Value") 0.0 ("Value") 0.0 ("Value")] -> w284
              tunnel: [64.0 ("Value") 0.5 ("Value") 1.0 ("Value")] -> w283
              frame "PWM" {
              }
              frame "Motor", Default {
              }
              frame "Analog Out" {
              }
            }
            n152 = property on="Motor" class="Clust (strict)"("Visible"=TRUE) -> ()  [unwired: 2 in, 2 out]
            n153 = property on="Value" class="Slide (strict)"("Value"=w284, "Scale.Minimum"=w286, "Scale.Maximum"=w285, "Scale.Increment"=w283) -> ()  [unwired: 2 in, 2 out]
            n154 = property on="On/Off" class="Bool (strict)"("Visible"=w288) -> ()  [unwired: 2 in, 2 out]
            n155 = property on="Test Slider" class="Slide (strict)"("Visible"=w288) -> ()  [unwired: 2 in, 2 out]
            n156 = property on="Test Ring" class="Ring (strict)"("Visible"=w288) -> ()  [unwired: 2 in, 2 out]
            n157 = property on="Rev/Fwd" class="Clust (strict)"("Visible"=w288) -> ()  [unwired: 2 in, 2 out]
          }
          frame "Servo" {
            w304 = FALSE ("Visible")
            n158 = call <vilib>:"NT Read Number.vi"("Name"=w306) -> ("Numeric"=w305:dbl)  [unwired: 9 in, 1 out]
            n159 = property on="Test Slider" class="Slide (strict)"("Visible"=TRUE, "Scale.Maximum"=170.0 ("Scale.Range:Maximum")) -> ()  [unwired: 2 in, 2 out]
            n160 = local write "Test Slider"(w305) -> ()
            n161 = property on="Motor" class="Clust (strict)"("Visible"=w304) -> ()  [unwired: 2 in, 2 out]
            n162 = property on="Rev/Fwd" class="Clust (strict)"("Visible"=w304) -> ()  [unwired: 2 in, 2 out]
            n163 = property on="On/Off" class="Bool (strict)"("Visible"=w304) -> ()  [unwired: 2 in, 2 out]
            n164 = property on="Test Ring" class="Ring (strict)"("Visible"=w304) -> ()  [unwired: 2 in, 2 out]
          }
          frame "Relay", "Solenoid" {
            w307 = FALSE ("Visible")
            n165 = property on="Motor" class="Clust (strict)"("Visible"=w307) -> ()  [unwired: 2 in, 2 out]
            n166 = property on="Test Slider" class="Slide (strict)"("Visible"=w307) -> ()  [unwired: 2 in, 2 out]
            n167 = Search and Replace String(input string=w308, search string="/Value  **", replace string="/Direction") -> (result string=w314:string)  [unwired: 5 in, 3 out]
            n168 = property on="Test Ring" class="Ring (strict)"("Visible"=w307) -> ()  [unwired: 2 in, 2 out]
            n169 = call <vilib>:"NT Read String.vi"("Name"=w314) -> ("String"=w312:string)  [unwired: 9 in, 1 out]
            n170 = Equal?(x="Both directions", y=w312) -> (x = y?=w310:bool)
            n171 = Not(x=w310) -> (.not. x?=w311:bool)
            n172 = property on="Rev/Fwd" class="Clust (strict)"("Visible"=w310) -> ()  [unwired: 2 in, 2 out]
            n173 = property on="On/Off" class="Bool (strict)"("Visible"=w311, "Caption.Text"=w309) -> ()  [unwired: 2 in, 2 out]
          }
          frame "Compressor", "Digital Out" {
            w317 = FALSE ("Visible")
            # "Get direction and finish"
            n174 = property on="Motor" class="Clust (strict)"("Visible"=w317) -> ()  [unwired: 2 in, 2 out]
            n175 = property on="Test Slider" class="Slide (strict)"("Visible"=w317) -> ()  [unwired: 2 in, 2 out]
            n176 = property on="Test Ring" class="Ring (strict)"("Visible"=w317) -> ()  [unwired: 2 in, 2 out]
            n177 = property on="On/Off" class="Bool (strict)"("Visible"=TRUE, "Caption.Text"=w318) -> ()  [unwired: 2 in, 2 out]
            n178 = property on="Rev/Fwd" class="Clust (strict)"("Visible"=FALSE) -> ()  [unwired: 2 in, 2 out]
          }
          frame "Camera" {
            n179 = call <vilib>:"Get Last Path Segment.vi"("String in"=w325) -> ("String out"=w326:string)  [unwired: 10 in]
            n180 = property on="On/Off" class="Bool (strict)"("Visible"=FALSE) -> ()  [unwired: 2 in, 2 out]
            n181 = property on="Motor" class="Clust (strict)"("Visible"=FALSE) -> ()  [unwired: 2 in, 2 out]
            n182 = property on="Rev/Fwd" class="Clust (strict)"("Visible"=FALSE) -> ()  [unwired: 2 in, 2 out]
            n183 = case shown="\"White Balance  **\"" w326 {
              tunnel: w325 -> [w332 w341 w350 w359 w368 _ w374]
              tunnel: w324 -> [w330 w338 w347 w356 w365 _ _]
              frame "Size  **" {
                n184 = Index Array(array=w330) -> (element=w329:cluster{string[]})  [unwired: 1 in]
                n185 = call <vilib>:"NT Read String.vi"("Name"=w332) -> ("String"=w331:string)  [unwired: 9 in, 1 out]
                n186 = Unbundle(w329) -> (w327:string[])
                n187 = Match First String(2:w327, 3:w331) -> (0:w328:i32)  [unwired: 1 out]
                n188 = property on="Test Ring" class="Ring (strict)"("Value"=w328, "Strings []"=w327) -> ()  [unwired: 2 in, 2 out]
                n189 = property on="Test Ring" class="Ring (strict)"("Visible"=TRUE) -> ()  [unwired: 2 in, 2 out]
                n190 = property on="Test Slider" class="Slide (strict)"("Visible"=FALSE) -> ()  [unwired: 2 in, 2 out]
              }
              frame "White Balance  **" {
                n191 = Index Array(array=w338, index=1) -> (element=w339:cluster{string[]})
                n192 = call <vilib>:"NT Read String.vi"("Name"=w341) -> ("String"=w340:string)  [unwired: 9 in, 1 out]
                n193 = Unbundle(w339) -> (w336:string[])
                n194 = Match First String(2:w336, 3:w340) -> (0:w335:i32)  [unwired: 1 out]
                n195 = property on="Test Ring" class="Ring (strict)"("Value"=w335, "Strings []"=w336) -> ()  [unwired: 2 in, 2 out]
                n196 = property on="Test Ring" class="Ring (strict)"("Visible"=TRUE) -> ()  [unwired: 2 in, 2 out]
                n197 = property on="Test Slider" class="Slide (strict)"("Visible"=FALSE) -> ()  [unwired: 2 in, 2 out]
              }
              frame "Exposure  **" {
                n198 = Index Array(array=w347, index=2) -> (element=w348:cluster{string[]})
                n199 = call <vilib>:"NT Read String.vi"("Name"=w350) -> ("String"=w349:string)  [unwired: 9 in, 1 out]
                n200 = Unbundle(w348) -> (w344:string[])
                n201 = Match First String(2:w344, 3:w349) -> (0:w345:i32)  [unwired: 1 out]
                n202 = property on="Test Ring" class="Ring (strict)"("Value"=w345, "Strings []"=w344) -> ()  [unwired: 2 in, 2 out]
                n203 = property on="Test Ring" class="Ring (strict)"("Visible"=TRUE) -> ()  [unwired: 2 in, 2 out]
                n204 = property on="Test Slider" class="Slide (strict)"("Visible"=FALSE) -> ()  [unwired: 2 in, 2 out]
              }
              frame "Exposure Priority  **" {
                n205 = Index Array(array=w356, index=3) -> (element=w357:cluster{string[]})
                n206 = call <vilib>:"NT Read String.vi"("Name"=w359) -> ("String"=w358:string)  [unwired: 9 in, 1 out]
                n207 = Unbundle(w357) -> (w353:string[])
                n208 = Match First String(2:w353, 3:w358) -> (0:w354:i32)  [unwired: 1 out]
                n209 = property on="Test Ring" class="Ring (strict)"("Value"=w354, "Strings []"=w353) -> ()  [unwired: 2 in, 2 out]
                n210 = property on="Test Ring" class="Ring (strict)"("Visible"=TRUE) -> ()  [unwired: 2 in, 2 out]
                n211 = property on="Test Slider" class="Slide (strict)"("Visible"=FALSE) -> ()  [unwired: 2 in, 2 out]
              }
              frame "Color Enable  **" {
                n212 = Index Array(array=w365, index=4) -> (element=w366:cluster{string[]})
                n213 = call <vilib>:"NT Read String.vi"("Name"=w368) -> ("String"=w367:string)  [unwired: 9 in, 1 out]
                n214 = Unbundle(w366) -> (w362:string[])
                n215 = Match First String(2:w362, 3:w367) -> (0:w363:i32)  [unwired: 1 out]
                n216 = property on="Test Ring" class="Ring (strict)"("Value"=w363, "Strings []"=w362) -> ()  [unwired: 2 in, 2 out]
                n217 = property on="Test Ring" class="Ring (strict)"("Visible"=TRUE) -> ()  [unwired: 2 in, 2 out]
                n218 = property on="Test Slider" class="Slide (strict)"("Visible"=FALSE) -> ()  [unwired: 2 in, 2 out]
              }
              frame Default {
                n219 = property on="Test Ring" class="Ring (strict)"("Visible"=FALSE) -> ()  [unwired: 2 in, 2 out]
                n220 = property on="Test Slider" class="Slide (strict)"("Visible"=FALSE) -> ()  [unwired: 2 in, 2 out]
              }
              frame "Brightness  **", "Color Level  **", "Compression  **", "FPS  **", "Sharpness  **" {
                n221 = call <vilib>:"NT Read Number.vi"("Name"=w374) -> ("Numeric"=w373:dbl)  [unwired: 9 in, 1 out]
                n222 = local write "Test Slider"(w373) -> ()
                n223 = property on="Test Slider" class="Slide (strict)"("Visible"=TRUE, "Scale.Maximum"=100.0 ("Scale.Range:Maximum")) -> ()  [unwired: 2 in, 2 out]
                n224 = property on="Test Ring" class="Ring (strict)"("Visible"=FALSE) -> ()  [unwired: 2 in, 2 out]
              }
            }
          }
        }
        n225 = property on="Progress" class="Clust (strict)"("Visible"=FALSE) -> ()  [unwired: 2 in, 2 out]
      }
      event "Test Name": Mouse Enter {
        # "Populate the ring with the list of tests"
        n226 = event-data() -> ()  [unwired: 1 in, 1 out]
        n227 = call <vilib>:"NT Read String Array.vi"("Name"="TestMode/TestList") -> ("String Array"=w382:string[])  [unwired: 9 in, 1 out]
        n228 = Build Array (concatenate)("Select the test to run...", w382) -> (w381:string[])
        n229 = property on="Test Name" class="Ring (strict)"("Strings []"=w381) -> ()  [unwired: 2 in, 2 out]
      }
      event "Test Name": Value Change {
        w384 = FALSE ("Visible")
        # "Tell the robot the test name to run"
        n230 = event-data() -> ("NewVal"=w388:u16)  [unwired: 1 in]
        n231 = property on="Test Name" class="Ring (strict)"() -> ("Strings []"=w389:string[])  [unwired: 2 in, 2 out]
        n232 = local write "Progress"(T7 {"Test Progress"=0, "Test Progress Text"=""} ("Progress")) -> ()
        n233 = Index Array(array=w389, index=w388) -> (element=w387:string)
        n234 = call <vilib>:"NT Write String.vi"("String"=w387, "Name"="TestMode/TestName") -> ()  [unwired: 9 in, 1 out]
        n235 = property on="Progress" class="Clust (strict)"("Visible"=TRUE) -> ()  [unwired: 2 in, 2 out]
        n236 = property on="Motor" class="Clust (strict)"("Visible"=w384) -> ()  [unwired: 2 in, 2 out]
        n237 = property on="Test Slider" class="Slide (strict)"("Visible"=w384) -> ()  [unwired: 2 in, 2 out]
        n238 = property on="On/Off" class="Bool (strict)"("Visible"=w384) -> ()  [unwired: 2 in, 2 out]
        n239 = property on="Rev/Fwd" class="Clust (strict)"("Visible"=w384) -> ()  [unwired: 2 in, 2 out]
        n240 = property on="Test Ring" class="Ring (strict)"("Visible"=w384) -> ()  [unwired: 2 in, 2 out]
      }
      event "Select Auto": Mouse Enter {
        # "Populate the combo box with the list of autonomous options"
        n241 = event-data() -> ()  [unwired: 1 in, 1 out]
        n242 = call <vilib>:"NT Read String Array.vi"("Name"="Auto List") -> ("String Array"=w391:string[])  [unwired: 9 in, 1 out]
        n243 = property on="Select Auto" class="CmbBox"("Strings[]"=w391) -> ()  [unwired: 2 in, 2 out]
      }
      event "Select Auto": Value Change {
        # "User modified the Auto Selection. Write to NT variable so robot knows."
        n244 = event-data() -> ("NewVal"=w394:string)  [unwired: 1 in]
        n245 = call <vilib>:"NT Write String.vi"("String"=w394, "Name"="Auto Selector") -> ()  [unwired: 9 in, 1 out]
      }
      event "Command Selection": Value Change {
        # "Get the params and show in table"
        n246 = event-data() -> ("NewVal"=w400:i32)  [unwired: 1 in]
        n247 = property on="Command Selection" class="MCListbox (strict)"() -> ("ItemNames"=w398:string[][])  [unwired: 2 in, 2 out]
        n248 = call <vilib>:"WPI_DashboardUpdate Command Params.vi"("NewVal"=w400, "Commands"=w398, "Param Tbl"=w399) -> ()  [unwired: 8 in, 1 out]
      }
      event "Execute Command": Value Change {
        # "Started one, Unique ID holds\nresponse"
        n249 = event-data() -> ()  [unwired: 1 in, 1 out]
        n250 = property on="Command Selection" class="MCListbox (strict)"() -> ("ItemNames"=w411:string[][])  [unwired: 2 in, 2 out]
        n251 = Index Array(array=w411, index (row)="Command Selection", index (col)=0) -> (element=w409:string)
        n252 = call <vilib>:"Invoke Commands.vi"("Command Params"="Command Params", "Function Name"=w409) -> ("Params"=w405:u8, "Started"=w404:bool)  [unwired: 7 in, 1 out]
        n253 = Array Subset(array="Command Params", length (row)=w405) -> (w406:string[][])  [unwired: 3 in]
        n254 = Select(t="Executing" ("Cmd Status"), s=w404, f="" ("Cmd Status")) -> (s? t:f=→"Cmd Status":string)
      }
      event "Command Selection": Double Click {
        n255 = event-data() -> ("Row"=w419:i32)  [unwired: 1 in]
        n256 = property on="Command Selection" class="MCListbox (strict)"() -> ("ItemNames"=w422:string[][])  [unwired: 2 in, 2 out]
        n257 = local read "Command Params"() -> (w418:string[][])
        n258 = Index Array(array=w422, index (row)=w419, index (col)=0) -> (element=w420:string)
        n259 = call <vilib>:"Invoke Commands.vi"("Command Params"=w418, "Function Name"=w420) -> ("Params"=w417:u8, "Started"=w412:bool)  [unwired: 7 in, 1 out]
        n260 = Array Subset(array=w418, length (row)=w417) -> (w416:string[][])  [unwired: 3 in]
        n261 = Select(t="Executing" ("Cmd Status"), s=w412, f="" ("Cmd Status")) -> (s? t:f=w413:string)
        n262 = local write "Cmd Status"(w413) -> ()
      }
      event "CheckList": Double Click {
        # "Shift clears all"
        # "Update symbols on the listbox"
        n263 = event-data() -> ("PlatMods.Shift"=w424:bool, "Row"=w426:i32)  [unwired: 1 in]
        n264 = case shown="True" w424 {
          tunnel: w426 -> [w430 _]
          tunnel: 1 -> [w429 _]
          frame False {
            n265 = property on="CheckList" class="LstBox (strict)"() -> ("Item Symbols"=w428:i32[])  [unwired: 2 in, 2 out]
            n266 = Replace Array Subset(array=w428, new element=w429, index=w430) -> (w427:i32[])
            n267 = property on="CheckList" class="LstBox (strict)"("Item Symbols"=w427) -> ()  [unwired: 2 in, 2 out]
          }
          frame True {
            w431 = 0 ("Top Row")
            n268 = property on="CheckList" class="LstBox (strict)"() -> ("Number of Rows"=w433:u32)  [unwired: 2 in, 2 out]
            n269 = Initialize Array(0, w433) -> (w432:i32[])
            n270 = property on="CheckList" class="LstBox (strict)"("Top Row"=w431, "Value"=w431, "Item Symbols"=w432) -> ()  [unwired: 2 in, 2 out]
          }
        }
      }
      event "CheckList": Key Down {
        # "Update symbols on the listbox\nLeft and right keys check and uncheck"
        n271 = event-data() -> ("VKey"=w437:T23)  [unwired: 1 in]
        n272 = case shown="\"Left\", \"Right\"" w437 {
          selector: w437 -> [w442 _]
          tunnel: eventvkey."Left" ("VKey") -> [w440 _]
          frame "Left", "Right" {
            n273 = Equal?(x=w440, y=w442) -> (x = y?=w441:bool)
            n274 = Select(t=0, s=w441, f=1) -> (s? t:f=w443:i32)
            n275 = property on="CheckList" class="LstBox (strict)"() -> ("Item Symbols"=w446:i32[])  [unwired: 2 in, 2 out]
            n276 = Replace Array Subset(array=w446, new element=w443, index="CheckList") -> (w445:i32[])
            n277 = property on="CheckList" class="LstBox (strict)"("Item Symbols"=w445) -> ()  [unwired: 2 in, 2 out]
          }
          frame Default {
          }
        }
      }
      event "Motor.Enable": Value Change {
        # "When the test mode otor enable helper is set, update that\ntree row item's value"
        n278 = event-data() -> ("NewVal"=w452:bool)  [unwired: 1 in]
        n279 = Unbundle("Motor") -> ("Value"=w451:dbl)  [unwired: 1 out]
        n280 = Select(t=w451, s=w452, f=0.0) -> (s? t:f=w449:dbl)
        n281 = call <vilib>:"NT Write Number.vi"("Numeric"=w449, "Name"=w448) -> ()  [unwired: 9 in, 1 out]
      }
      event "Test Slider": Value Change {
        # "When the test mode slider helper is set, update that\ntree row item's value"
        n282 = event-data() -> ("NewVal"=w455:dbl)  [unwired: 1 in]
        n283 = call <vilib>:"NT Write Number.vi"("Numeric"=w455, "Name"=w456) -> ()  [unwired: 9 in, 1 out]
      }
      event "On/Off": Value Change {
        # "When the test mode on/off helper value is set, update that\ntree row item's value"
        n284 = event-data() -> ("NewVal"=w460:bool)  [unwired: 1 in]
        n285 = Boolean To (0,1)(Boolean=w460) -> (0, 1=w459:i16)
        n286 = call <vilib>:"NT Write Number.vi"("Numeric"=w459, "Name"=w458) -> ()  [unwired: 9 in, 1 out]
      }
      event "Rev/Fwd": Value Change {
        # "When the test mode helper value for relays is set, update that\ntree row item's value"
        n287 = event-data() -> ("NewVal.Forward"=w468:bool, "NewVal.Reverse"=w467:bool)  [unwired: 1 in]
        n288 = Boolean To (0,1)(Boolean=w468) -> (0, 1=w464:i16)
        n289 = Boolean To (0,1)(Boolean=w467) -> (0, 1=w466:i16)
        n290 = Negate(x=w466) -> (-x=w465:i16)
        n291 = Add(x=w464, y=w465) -> (x+y=w463:i16)
        n292 = call <vilib>:"NT Write Number.vi"("Numeric"=w463, "Name"=w462) -> ()  [unwired: 9 in, 1 out]
      }
      event "Test Ring": Value Change {
        # "When a test mode helper value is selected from the ring,\nset the tree item's variable to the string value"
        n293 = event-data() -> ("NewVal"=w472:u16)  [unwired: 1 in]
        n294 = property on="Test Ring" class="Ring (strict)"() -> ("Strings []"=w473:string[])  [unwired: 2 in, 2 out]
        n295 = Index Array(array=w473, index=w472) -> (element=w471:string)
        n296 = call <vilib>:"NT Write String.vi"("String"=w471, "Name"=w470) -> ()  [unwired: 9 in, 1 out]
      }
      event "Rec Mode": Value Change {
        # "Update globals for recording mode and path to read log from.\nClear when logging and let NetworkTables set path for vision to\nuse."
        n297 = event-data() -> ("NewVal"=w484:enum32{"Stop", "Record", "Playback"})  [unwired: 1 in]
        n298 = global write "WPI_DashboardLogging Global.vi" "Logging Filename"(path "") -> ()
        n299 = global write "WPI_DashboardLogging Global.vi" "Recording"(w484) -> ()
        n300 = case shown="\"Playback\"" w484 {
          tunnel: w483 -> [_ w486 w495]
          tunnel: [_ _ w494] -> w481
          tunnel: [_ _ w493] -> _
          tunnel: w479 -> [_ _ w491]
          tunnel: cluster{i32, i32} {-250, 170} -> [_ _ w490]
          tunnel: [_ _ T24 {"Image Size"=TRUE, "Image Type"=TRUE, "Pixel Value"=TRUE, "ROI Information"=TRUE, "Zoom Factor"=FALSE} ("Image Information Shown:All Elements")] -> w474
          tunnel: [_ _ TRUE ("Zoom Factor")] -> w475
          tunnel: w477 -> [_ _ w487]
          frame Default {
          }
          frame "Stop", "Record" {
            # "Place Window too"
            n301 = invoke class="VI" method="FP.Close"(reference=w486) -> (reference out=w485:refnum<vi>)  [unwired: 2 in, 2 out]
            n302 = invoke class="VI" method="Abort VI"(reference=w485) -> ()  [unwired: 2 in, 3 out]
          }
          frame "Playback" {
            n303 = call "Open Playback Panel.vi"("Offset"=w490, "DB VI Ref"=w491, "Playback in"=w495) -> ("Playback out"=w492:refnum<vi>)  [unwired: 8 in]
            n304 = register-events(w492, w487) -> (reference out=w494:refnum<event-registration>, error out=w493:errorcluster)  [unwired: 2 in]
          }
        }
        n305 = property on="Camera Image Right" class="ImageControl"("Image Information Shown"=w474, "Image Information Visible"=w475) -> ()  [unwired: 2 in, 2 out]
        n306 = property on="Camera Image" class="ImageControl"("Image Information Shown"=w474, "Image Information Visible"=w475) -> ()  [unwired: 2 in, 2 out]
        n307 = call <vilib>:"WPI_DashboardNT Log FieldName Cache.vi"("Operation"=enum16{"Lookup/Add", "Index", "Clear"}."Clear") -> ()  [unwired: 8 in, 3 out]
      }
      event Panel Close {
        w497 = enum32{"Stop", "Record", "Playback"}."Stop" ("Rec Mode")
        # "Playback window has been closed, abort"
        n308 = event-data() -> ()  [unwired: 1 in, 4 out]
        n309 = local write "Rec Mode"(w497) -> ()
        n310 = global write "WPI_DashboardLogging Global.vi" "Recording"(w497) -> ()
      }
      event Panel Close {
        # "Abort playback window and ourself"
        n311 = event-data() -> ()  [unwired: 1 in, 4 out]
        n312 = invoke class="VI" method="FP.Close"(reference=w501) -> (reference out=w500:refnum<vi>)  [unwired: 2 in, 2 out]
        n313 = invoke class="VI" method="Abort VI"(reference=w500) -> (error out=w499:errorcluster)  [unwired: 2 in, 2 out]
        n314 = invoke class="VI" method="Abort VI"(error in=w499) -> ()  [unwired: 2 in, 3 out]
      }
      event User Event {
        n315 = event-data() -> ("IDs"=w508:cluster{"RPC field ID":u16, "Unique ID":u16}, "String"=w507:string)  [unwired: 1 in]
        n316 = Bundle("IDs"=w508, "String"=w507) -> (w506:T10)  [unwired: 1 in]
        n317 = call <vilib>:"Retrieve RPC Response.vi"("RPC Response"=w506) -> ("Output"=w504:string[][])  [unwired: 10 in]
        n318 = Build Array (concatenate)(w502, w504) -> (w503:string[][])
        n319 = local write "Command Params"(w503) -> ()
        n320 = local write "Cmd Status"("" ("Cmd Status")) -> ()
      }
      event "Tree": Double Click {
        n321 = event-data() -> ("PlatMods"=w514:T27, "Tag"=w511:string)  [unwired: 1 in]
        n322 = Unbundle(w514) -> ("Shift"=w513:bool)  [unwired: 4 out]
        n323 = String Subset(string=w511, length (rest)=1 ("length (rest)")) -> (substring=w510:string)  [unwired: 1 in]
        n324 = Not(x=w513) -> (.not. x?=w512:bool)
        n325 = case shown="\"/\"" w510 {
          tunnel: w511 -> [_ w517]
          tunnel: w512 -> [_ w516]
          frame Default {
          }
          frame "/" {
            n326 = call <vilib>:"NT Update Persistence.vi"("Persistence"=w516, "Name"=w517) -> ()  [unwired: 9 in, 1 out]
          }
        }
      }
    }
  }
  n327 = while {
    tunnel: w65 -> [w519]
    i -> [w522]
    stop <- FALSE stop-if-true
    n328 = Wait (ms)(milliseconds to wait=u32 100) -> ()  [unwired: 1 out]
    n329 = case shown="\"Playback\"" "Rec Mode" {
      tunnel: w522 -> [_ _ w537]
      tunnel: [u32 2829099 ("Base Color") u32 11141120 ("Target Color") w526] -> w518
      frame "Stop", Default {
        # "Reset the color, extra updates don't cost much"
      }
      frame "Record" {
      }
      frame "Playback" {
        # "Playback"
        n330 = Quotient & Remainder(x=w537, y=u32 50 ("milliseconds to wait")) -> (x-y*floor(x/y)=w533:u32)  [unwired: 1 out]
        n331 = Divide(x=w533, y=u32 50 ("milliseconds to wait")) -> (x/y=w530:dbl)
        n332 = Multiply(x=6.283185307179586, y=w530) -> (x*y=w535:dbl)
        n333 = Sine(x=w535) -> (sin(x)=w534:dbl)
        n334 = Absolute Value(x=w534) -> (abs(x)=w527:dbl)
        n335 = call "Interpolate RGB Color.vi"("Proportion"=w527, "Target Color"=u32 30976, "Base Color"=u32 2829099) -> ("Result Color"=w526:u32)  [unwired: 8 in]
      }
    }
    n336 = property class="Pane"(reference=w519, "PaneColor"=w518) -> ()  [unwired: 1 in, 2 out]
  }
  n337 = local write "Dashboard Tab"(T3."Drive" ("Dashboard Tab")) -> ()
  n338 = property on="On/Off" class="Bool (strict)"("Visible"=w36) -> ()  [unwired: 2 in, 2 out]
  n339 = property on="Motor" class="Clust (strict)"("Visible"=w36) -> ()  [unwired: 2 in, 2 out]
  n340 = property on="Progress" class="Clust (strict)"("Visible"=w36) -> ()  [unwired: 2 in, 2 out]
  n341 = property on="Test Ring" class="Ring (strict)"("Visible"=w36) -> ()  [unwired: 2 in, 2 out]
  n342 = property on="Rev/Fwd" class="Clust (strict)"("Visible"=w36) -> ()  [unwired: 2 in, 2 out]
  n343 = while {
    tunnel: u16 1741 ("timeout ms (25000)") -> [w539]
    stop <- FALSE stop-if-true
    n344 = TCP Create Listener(10:w539) -> (0:w538:errorcluster, 3:w540:refnum<k5>)  [unwired: 4 in, 1 out]
    n345 = case shown="No Error" w538 {
      selector: w538 -> [w542 _]
      tunnel: w540 -> [w543 _]
      frame No Error {
        n346 = while {
          tunnel: w543 -> [w546]
          tunnel: w542 -> [w545]
          stop <- FALSE stop-if-true
          n347 = TCP Wait On Listener(8:w545, 11:w546) -> (0:w547:errorcluster, 4:w548:refnum<k5>)  [unwired: 2 in, 3 out]
          n348 = local write "TCP"(w548) -> ()
          n349 = case shown="No Error" w547 {
            frame No Error {
            }
            frame Error {
              n350 = Wait (ms)(milliseconds to wait=u32 1000) -> ()  [unwired: 1 out]
            }
          }
        }
      }
      frame Error {
        n351 = Wait (ms)(milliseconds to wait=u32 1000) -> ()  [unwired: 1 out]
      }
    }
  }
  n352 = local write "Command Selection"(u16 0 ("milliseconds to wait")) -> ()
  n353 = local write "Command Params"(string[][] [] ("Command Params")) -> ()
  n354 = global write "WPI_DashboardLogging Global.vi" "Recording"(w59) -> ()
  n355 = local write "Rec Mode"(w59) -> ()
  n356 = call <vilib>:"NT Write String.vi"("String"="Select Auto", "Name"="Auto Selector") -> ()  [unwired: 9 in, 1 out]
